vi "Utilities_Justify Text Position.vi"(5 "Final Size":i32, 7 "Max Width":i32, 8 "Error":errorcluster, 10 "Justify":T1, 11 "Postion":T2) -> (0 "Error Out":errorcluster, 3 "Position Out":T2)   [LabVIEW 2014]
doc: "Set a new position based on the Justify input"
uses:
  Controls/Cluster/Cluster_Top Left position.ctl
  Controls/Enum/ENUM_Text Justify.ctl
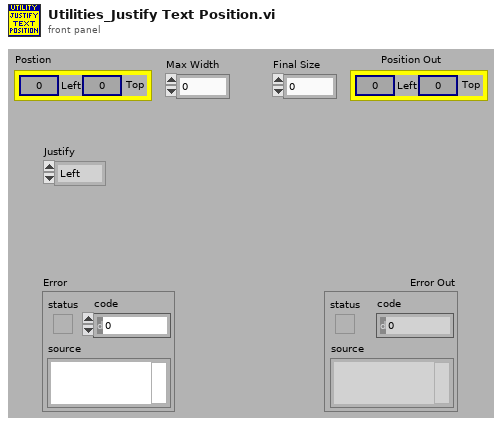
[diagram p1: front panel]
types:
  T1 = typedef "ENUM_Text Justify.ctl" = enum16{"Left", "Center", "Right"}
  T2 = typedef "Cluster_Top Left position.ctl" = cluster{"Left":i32, "Top":i32}
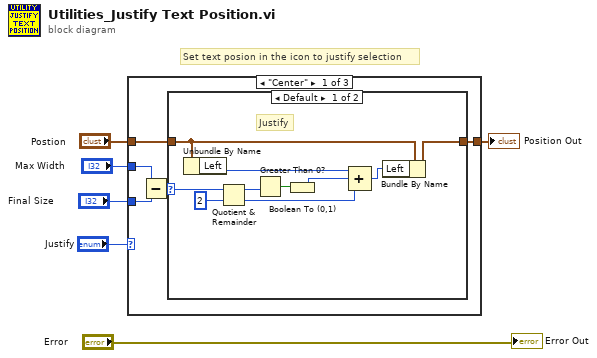
[diagram p0: block diagram]
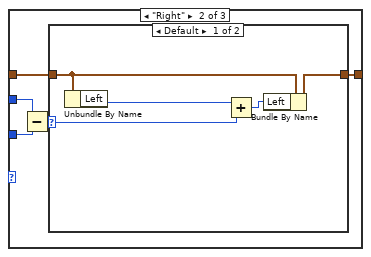
[diagram p3: hidden frame]
diagram:
  # "Set text posion in the icon to justify selection"
  n1 = case shown="\"Center\"" "Justify" {
    tunnel: "Max Width" -> [w11 w27 _]
    tunnel: "Final Size" -> [w10 w26 _]
    tunnel: "Postion" -> [w8 w24 w34]
    tunnel: [w7 w23 w34] -> w3
    frame "Center" {
      n2 = Subtract(x=w11, y=w10) -> (x-y=w9:i32)
      n3 = case shown="Default" w9 {
        selector: w9 -> [w21 _]
        tunnel: w8 -> [w19 w22]
        tunnel: [w16 w22] -> w7
        frame Default {
          # "Justify"
          n4 = Unbundle By Name(w19) -> ("Left"=w17:i32)
          n5 = Quotient & Remainder(x=w21, y=2) -> (x-y*floor(x/y)=w15:i32, floor(x/y)=w13:i32)
          n6 = Greater Than 0?(x=w15) -> (x > 0?=w14:bool)
          n7 = Boolean To (0,1)(Boolean=w14) -> (0, 1=w12:i16)
          n8 = Compound Arithmetic op=ADD(w17, w12, w13) -> (w18:i32)
          n9 = Bundle By Name(cluster=w19, "Left"=w18) -> (w16:T2)
        }
        frame ..1 {
        }
      }
    }
    frame "Right" {
      n10 = Subtract(x=w27, y=w26) -> (x-y=w25:i32)
      n11 = case shown="Default" w25 {
        selector: w25 -> [w28 _]
        tunnel: w24 -> [w32 w33]
        tunnel: [w29 w33] -> w23
        frame Default {
          n12 = Unbundle By Name(w32) -> ("Left"=w30:i32)
          n13 = Add(x=w30, y=w28) -> (x+y=w31:i32)
          n14 = Bundle By Name(cluster=w32, "Left"=w31) -> (w29:T2)
        }
        frame ..0 {
        }
      }
    }
    frame "Left" {
    }
  }
  "Position Out" <- w3
  "Error Out" <- "Error"
